vi "Open Connection.vi"(8 "error in (no error)":errorcluster, 10 "BAUD":u16, 11 "Port":string) -> (0 "error out":errorcluster, 3 "MB class out":refnum<class "MB class.lvclass">)   [LabVIEW 2020, in "MB class.lvclass"]
uses:
  MB class.lvclass
  MB class.lvclass/MB class.ctl
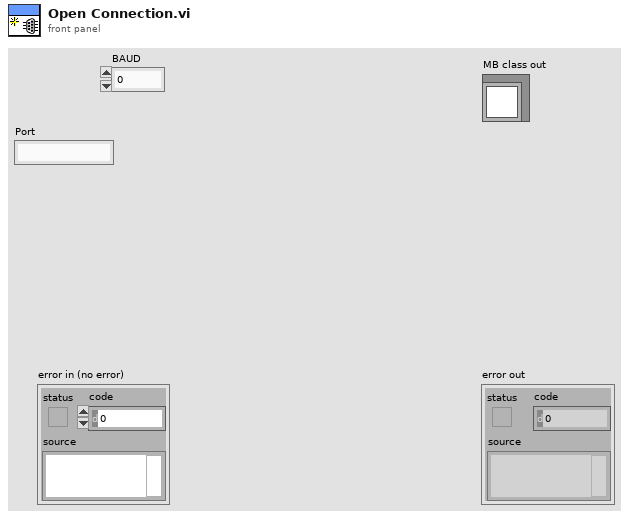
[diagram p1: front panel]
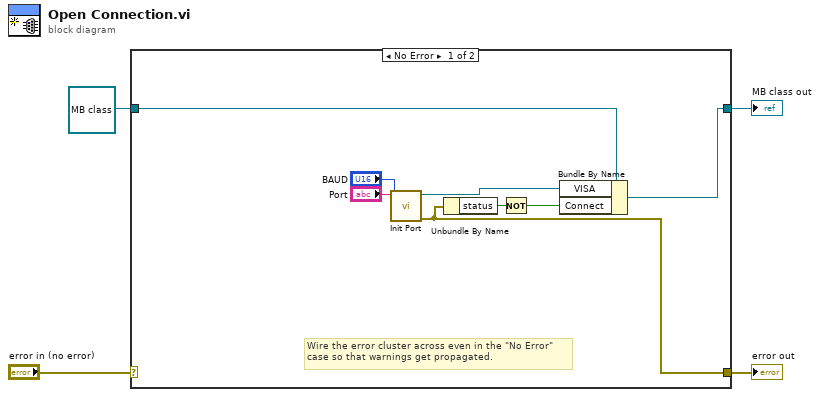
[diagram p0: block diagram]
diagram:
  n1 = case shown="No Error" "error in (no error)" {
    selector: "error in (no error)" -> [_ w14]
    tunnel: [w7 w14] -> w3
    tunnel: [w10 w13] -> w1
    tunnel: refnum<class "MB class.lvclass"> refnum ("MB class in") -> [w11 w13]
    frame No Error {
      # "Wire the error cluster across even in the \"No Error\"\ncase so that warnings get propagated."
      n2 = call "Init Port.vi"("BAUD"="BAUD", "String"="Port") -> ("error out"=w7:errorcluster, "VISA Refnum out"=w12:refnum<visa-resource-name>)  [unwired: 8 in]
      n3 = Unbundle By Name(w7) -> ("status"=w6:bool)
      n4 = Not(x=w6) -> (.not. x?=w5:bool)
      n5 = Bundle By Name(cluster=w11, "VISA"=w12, "Connect"=w5) -> (w10:refnum<class "MB class.lvclass">)
    }
    frame Error {
    }
  }
  "error out" <- w3
  "MB class out" <- w1
